vi "Actor Core.vi"(8 "error in":errorcluster, 11 "Philosopher in":refnum<class "Philosopher.lvclass">) -> (0 "error out":errorcluster, 3 "Philosopher out":refnum<class "Actor.lvclass">)   [LabVIEW 2023, in "Philosopher.lvlib" / "Philosopher.lvclass"]
uses:
  Philosopher.lvclass
  <vilib>/ActorFramework/Actor/Actor.lvclass
  Philosopher.lvclass/Philosopher.ctl
panel:
  out "ID":i32
  out "State Picture":u16(ring)
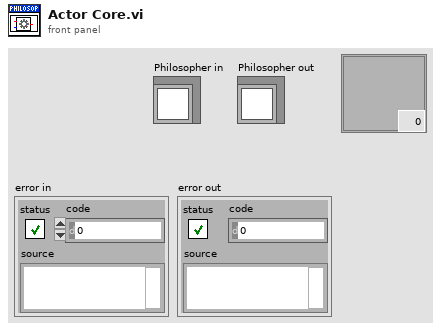
[diagram p1: front panel]
types:
  T1 = enum32{"Invalid", "Standard", "Closed", "Hidden", "Minimized", "Maximized"}
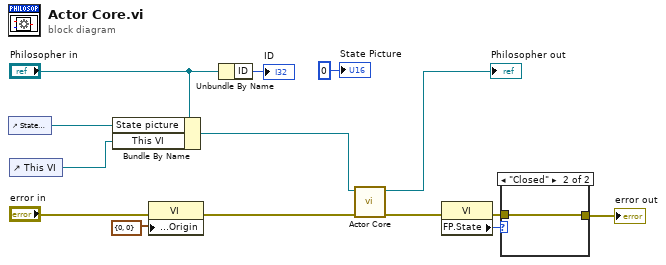
[diagram p0: block diagram]
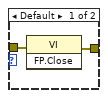
[diagram p2: hidden frame]
diagram:
  n1 = control-ref of="State Picture"() -> (w2:refnum<vi>)
  n2 = control-ref of="This VI"() -> (w11:refnum<vi>)
  n3 = Bundle By Name(cluster="Philosopher in", "State picture"=w2, "This VI"=w11) -> (w10:refnum<class "Philosopher.lvclass">)
  n4 = property class="VI"(error in="error in", "Front Panel Window:Origin"=cluster{"Horizontal":i16, "Vertical":i16} {"Horizontal"=0, "Vertical"=0}) -> (error out=w7:errorcluster)  [unwired: 1 in, 1 out]
  n5 = Unbundle By Name("Philosopher in") -> ("ID"=→"ID":i32)
  n6 = call-parent "Actor Core.vi"("error in"=w7, "Actor in"=w10) -> ("error out"=w4:errorcluster, "Actor out"=→"Philosopher out":refnum<class "Actor.lvclass">)  [unwired: 8 in]
  n7 = property on="Property Node" class="VI"(error in=w4) -> (error out=w5:errorcluster, "FP.State"=w6:T1)  [unwired: 1 in, 1 out]
  n8 = case shown="\"Closed\"" w6 {
    tunnel: w5 -> [w16 w17]
    tunnel: [w15 w17] -> w3
    frame Default {
      n9 = invoke class="VI" method="FP.Close"(error in=w16) -> (error out=w15:errorcluster)  [unwired: 2 in, 2 out]
    }
    frame "Closed" {
    }
  }
  "error out" <- w3
  "State Picture" <- u16 0 ("State Picture")
